vi "Anritsu VNA Read External Trigger Mode.vi"(7 "Anritsu VNA":T1, 8 "error in (no error)":errorcluster, 11 "VISA Resource Name":refnum<visa-resource-name>) -> (0 "error out":errorcluster, 2 "Ext. Trigger Mode":T2, 3 "dup VISA Resource Name":refnum<visa-resource-name>)   [LabVIEW 2011]
doc: "This VI for the HP8753B Network Analyzers reads the stimulus values. Except when performing log sweeps and freq list sweeps, this VI uses the start and stop values and the number of points to calcuate the stimulus values."
uses:
  TypeDefs/Anritsu VNA External Trigger Mode.ctl
  TypeDefs/Anritsu VNA Instrument Info.ctl
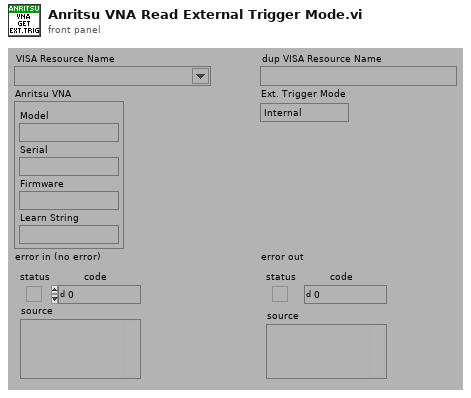
[diagram p1: front panel]
types:
  T1 = typedef "Anritsu VNA Instrument Info.ctl" = cluster{"Model":string, "Serial":string, "Firmware":string, "Learn String":string}
  T2 = typedef "Anritsu VNA External Trigger Mode.ctl" = enum16{"Internal", "External", "Manual", "GPIB"}
  T3 = typedef "Anritsu VNA Model.ctl" = enum16{"Not Supported", "37XXXX", "MS20XXX", "MS462XX", "MS464XX"}
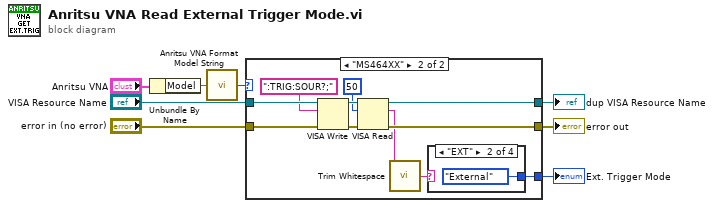
[diagram p0: block diagram]
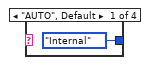
[diagram p3: hidden frame]
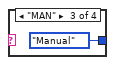
[diagram p4: hidden frame]
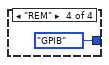
[diagram p5: hidden frame]
diagram:
  n1 = Unbundle By Name("Anritsu VNA") -> ("Model"=w1:string)
  n2 = call "Anritsu VNA Format Model String.vi"("Model"=w1) -> ("Model"=w3:T3)
  n3 = case shown="\"MS464XX\"" w3 {
    tunnel: "error in (no error)" -> [w9 w17]
    tunnel: [w9 w16] -> w7
    tunnel: "VISA Resource Name" -> [w10 w18]
    tunnel: [w10 w15] -> w5
    tunnel: [_ w11] -> w4
    frame "Not Supported".."MS462XX" {
    }
    frame "MS464XX" {
      n4 = VISA Write(VISA resource name=w18, write buffer=":TRIG:SOUR?;", error in (no error)=w17) -> (VISA resource name out=w21:refnum<visa-resource-name>, error out=w20:errorcluster)  [unwired: 1 out]
      n5 = VISA Read(VISA resource name=w21, byte count=u32 50, error in (no error)=w20) -> (VISA resource name out=w15:refnum<visa-resource-name>, read buffer=w13:string, error out=w16:errorcluster)  [unwired: 1 out]
      n6 = call <vilib>:"Trim Whitespace.vi"("string"=w13) -> ("trimmed string"=w12:string)  [unwired: 1 in]
      n7 = case shown="\"EXT\"" w12 {
        tunnel: [Anritsu_VNA_External_Trigger_Mode."Internal" Anritsu_VNA_External_Trigger_Mode."External" Anritsu_VNA_External_Trigger_Mode."Manual" Anritsu_VNA_External_Trigger_Mode."GPIB"] -> w11
        frame "AUTO", Default {
        }
        frame "EXT" {
        }
        frame "MAN" {
        }
        frame "REM" {
        }
      }
    }
  }
  "dup VISA Resource Name" <- w5
  "error out" <- w7
  "Ext. Trigger Mode" <- w4
